vi "Signal Generation.vi"() -> ()   [LabVIEW 2015]
uses:
  <vilib>/measure/NI_MABase.lvlib
panel:
  in  "Signal Repeats?":i32
  out "Waveform Chart":waveform(dbl)(graph)
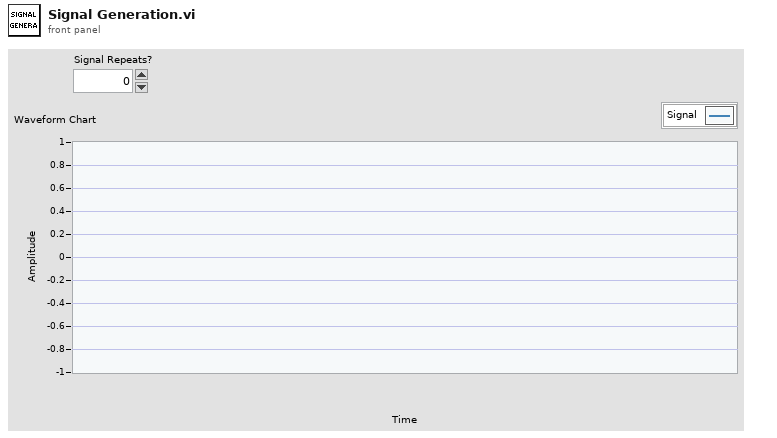
[diagram p1: front panel]
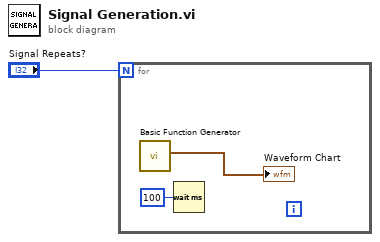
[diagram p0: block diagram]
diagram:
  n1 = for {
    N: "Signal Repeats?" -> [_]
    n2 = call <vilib>:"Basic Function Generator.vi"() -> ("signal out"=→"Waveform Chart":waveform(dbl))  [unwired: 9 in, 2 out]
    n3 = Wait (ms)(milliseconds to wait=u32 100) -> ()  [unwired: 1 out]
  }
